vi "Untitled 8 (SubVI).vi"(8 "error in (no error)":errorcluster, 11 "TreeControl in":refnum<vi>) -> (0 "error out":errorcluster, 3 "Setup out":refnum<class "Setup.lvclass">)   [LabVIEW 2013, in "DataCreation.lvlib"]
uses:
  DataCreation.lvlib
  classes/Datastructure/Setup/Setup.lvclass
  classes/Datastructure/Image/img.lvclass
  classes/Datastructure/Device/Device.lvclass
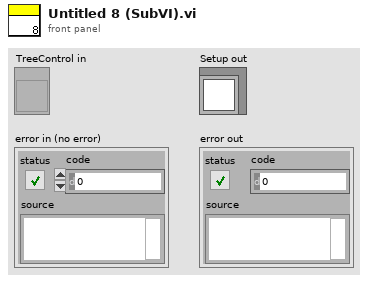
[diagram p1: front panel]
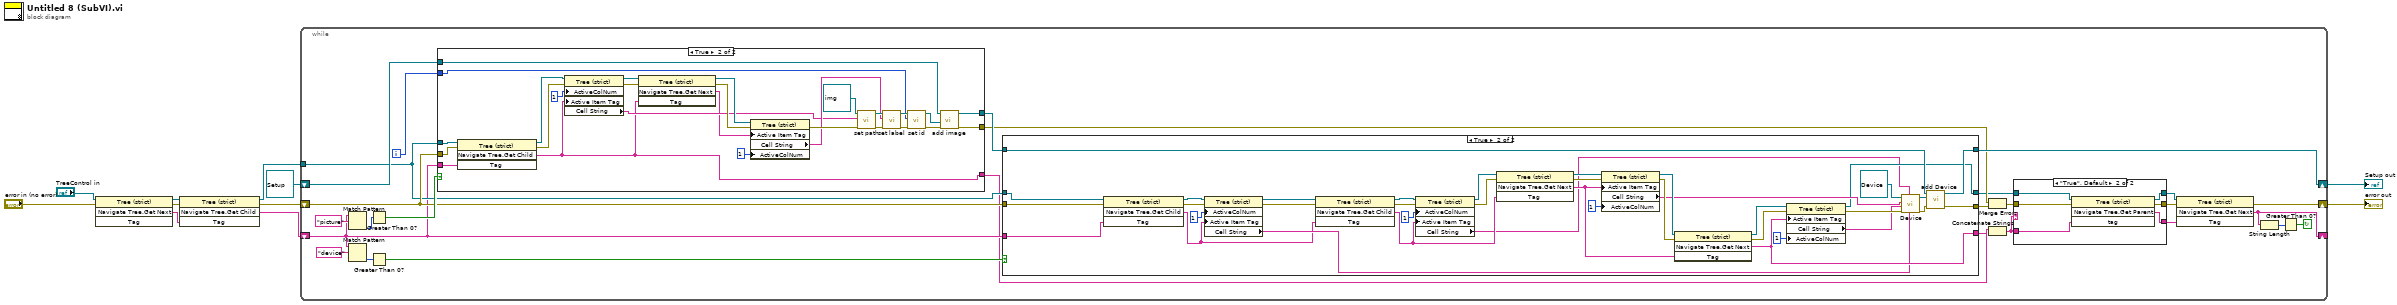
[diagram p0: block diagram]
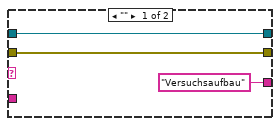
[diagram p2: hidden frame]
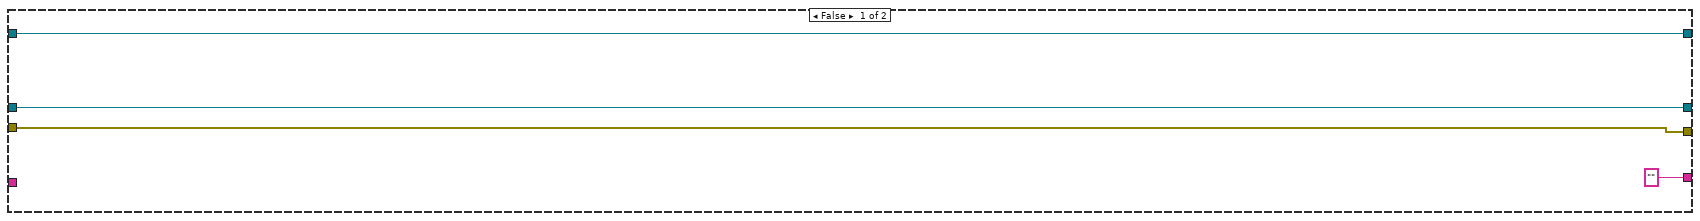
[diagram p3: hidden frame]
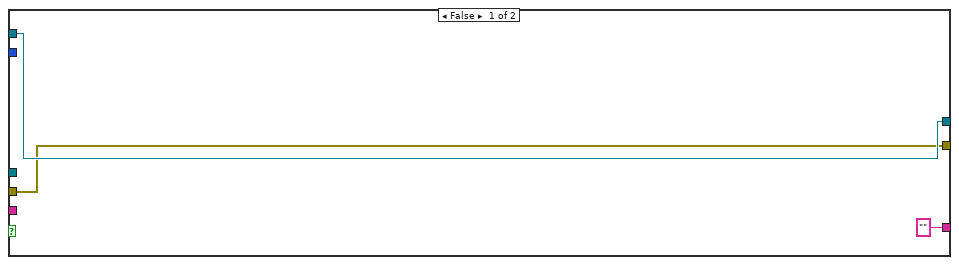
[diagram p4: hidden frame]
diagram:
  n1 = invoke class="Tree (strict)" method="Navigate Tree.Get Next"(reference="TreeControl in", error in="error in (no error)") -> (reference out=w5:refnum<vi>, error out=w6:errorcluster, "Navigate Tree:Get Next Item"=w7:string)  [unwired: 2 in, 1 out]
  n2 = invoke class="Tree (strict)" method="Navigate Tree.Get Child"(reference=w5, error in=w6, "Tag"=w7) -> (reference out=w10:refnum<vi>, error out=w8:errorcluster, "Navigate Tree:Get Child"=w9:string)  [unwired: 1 in, 1 out]
  n3 = while {
    shift-right: [w16] -> w1
    shift-left: w8 -> [w32]
    shift-right: [w25] -> w2
    shift-left: refnum<class "Setup.lvclass"> refnum ("Setup Ausgang") -> [w31]
    shift-right: [w14] -> _
    shift-left: w9 -> [w29]
    tunnel: w10 -> [w30]
    i -> [w12]
    stop <- w19 continue-if-true
    n4 = Match Pattern(string=w29, regular expression="picture" ("Regulärer Ausdruck")) -> (offset past match=w37:i32)  [unwired: 1 in, 3 out]
    n5 = Match Pattern(string=w29, regular expression="device" ("Regulärer Ausdruck")) -> (offset past match=w33:i32)  [unwired: 1 in, 3 out]
    n6 = Greater Than 0?(x=w37) -> (x > 0?=w36:bool)
    n7 = Greater Than 0?(x=w33) -> (x > 0?=w35:bool)
    n8 = case shown="True" w36 {
      tunnel: w29 -> [_ w99]
      tunnel: w32 -> [w89 w100]
      tunnel: w30 -> [_ w101]
      tunnel: [w89 w105] -> w24
      tunnel: w31 -> [w90 w104]
      tunnel: [w90 w98] -> w26
      tunnel: ["" ("Navigate Tree:Get Child") w97] -> w28
      tunnel: w12 -> [_ w94]
      frame False {
      }
      frame True {
        n9 = invoke class="Tree (strict)" method="Navigate Tree.Get Child"(reference=w101, error in=w100, "Tag"=w99) -> (reference out=w103:refnum<vi>, error out=w102:errorcluster, "Navigate Tree:Get Child"=w97:string)  [unwired: 1 in, 1 out]
        n10 = property class="Tree (strict)"(reference=w103, error in=w102, "ActiveColNum"=1 ("Active Cell:Active Column Number"), "Active Item Tag"=w97) -> (reference out=w113:refnum<vi>, error out=w114:errorcluster, "Cell String"=w109:string)
        n11 = invoke class="Tree (strict)" method="Navigate Tree.Get Next"(reference=w113, error in=w114, "Tag"=w97) -> (reference out=w112:refnum<vi>, error out=w111:errorcluster, "Navigate Tree:Get Next Item"=w108:string)  [unwired: 1 in, 1 out]
        n12 = property class="Tree (strict)"(reference=w112, error in=w111, "Active Item Tag"=w108, "ActiveColNum"=1 ("Active Cell:Active Column Number")) -> (error out=w118:errorcluster, "Cell String"=w110:string)  [unwired: 1 out]
        n13 = call-dynamic "set path.vi"("error in (no error)"=w118, "path"=w109, "img (Eingang)"=refnum<class "img.lvclass"> refnum ("img.lvclass")) -> ("error out"=w117:errorcluster, "img (Ausgang)"=w115:refnum<class "img.lvclass">)  [unwired: 7 in]
        n14 = call-dynamic "set label.vi"("error in (no error)"=w117, "label"=w110, "img (Eingang)"=w115) -> ("error out"=w95:errorcluster, "img (Ausgang)"=w96:refnum<class "img.lvclass">)  [unwired: 7 in]
        n15 = call-dynamic "set id.vi"("error in (no error)"=w95, "id"=w94, "img in"=w96) -> ("error out"=w93:errorcluster, "img out"=w92:refnum<class "img.lvclass">)  [unwired: 7 in]
        n16 = call-dynamic "add image.vi"("error in (no error)"=w93, "img.lvclass"=w92, "Setup (Eingang)"=w104) -> ("error out"=w105:errorcluster, "Setup (Ausgang)"=w98:refnum<class "Setup.lvclass">)  [unwired: 7 in]
      }
    }
    n17 = case shown="True" w35 {
      tunnel: w32 -> [w49 w53]
      tunnel: w30 -> [w48 w52]
      tunnel: w29 -> [_ w54]
      tunnel: ["" ("Navigate Tree:Get Next Item") w72] -> w27
      tunnel: w26 -> [w50 w66]
      tunnel: [w49 w67] -> w23
      tunnel: [w50 w65] -> w25
      tunnel: [w48 w64] -> w21
      frame False {
      }
      frame True {
        n18 = invoke class="Tree (strict)" method="Navigate Tree.Get Child"(reference=w52, error in=w53, "Tag"=w54) -> (reference out=w61:refnum<vi>, error out=w60:errorcluster, "Navigate Tree:Get Child"=w55:string)  [unwired: 1 in, 1 out]
        n19 = property class="Tree (strict)"(reference=w61, error in=w60, "ActiveColNum"=1 ("Active Cell:Active Column Number"), "Active Item Tag"=w55) -> (reference out=w57:refnum<vi>, error out=w58:errorcluster, "Cell String"=w56:string)
        n20 = invoke class="Tree (strict)" method="Navigate Tree.Get Child"(reference=w57, error in=w58, "Tag"=w55) -> (reference out=w81:refnum<vi>, error out=w82:errorcluster, "Navigate Tree:Get Child"=w80:string)  [unwired: 1 in, 1 out]
        n21 = property class="Tree (strict)"(reference=w81, error in=w82, "ActiveColNum"=1 ("Active Cell:Active Column Number"), "Active Item Tag"=w80) -> (reference out=w87:refnum<vi>, error out=w88:errorcluster, "Cell String"=w62:string)
        n22 = invoke class="Tree (strict)" method="Navigate Tree.Get Next"(reference=w87, error in=w88, "Tag"=w80) -> (reference out=w86:refnum<vi>, error out=w85:errorcluster, "Navigate Tree:Get Next Item"=w73:string)  [unwired: 1 in, 1 out]
        n23 = property class="Tree (strict)"(reference=w86, error in=w85, "Active Item Tag"=w73, "ActiveColNum"=1 ("Active Cell:Active Column Number")) -> (reference out=w78:refnum<vi>, error out=w79:errorcluster, "Cell String"=w74:string)
        n24 = invoke class="Tree (strict)" method="Navigate Tree.Get Next"(reference=w78, error in=w79, "Tag"=w73) -> (reference out=w77:refnum<vi>, error out=w76:errorcluster, "Navigate Tree:Get Next Item"=w72:string)  [unwired: 1 in, 1 out]
        n25 = property class="Tree (strict)"(reference=w77, error in=w76, "Active Item Tag"=w72, "ActiveColNum"=1 ("Aktive Zelle:Nummer der aktiven Spalte")) -> (reference out=w64:refnum<vi>, error out=w71:errorcluster, "Cell String"=w63:string)
        n26 = call-dynamic "Device.vi"("Model"=w56, "last calibration"=w62, "error in (no error)"=w71, "Hersteller"=w63, "serial"=w74, "Device Eingang"=refnum<class "Device.lvclass"> refnum ("Device.lvclass")) -> ("error out"=w68:errorcluster, "Device Ausgang"=w69:refnum<class "Device.lvclass">)  [unwired: 4 in]
        n27 = call-dynamic "add Device.vi"("error in (no error)"=w68, "Device.lvclass"=w69, "Setup Eingang"=w66) -> ("error out"=w67:errorcluster, "Setup Ausgang"=w65:refnum<class "Setup.lvclass">)  [unwired: 7 in]
      }
    }
    n28 = Merge Errors(w24, w23) -> (w22:errorcluster)
    n29 = Concatenate Strings(w28, w27) -> (w13:string)
    n30 = case shown="\"True\", Default" w13 {
      tunnel: w22 -> [w41 w47]
      tunnel: w21 -> [w40 w46]
      tunnel: w13 -> [_ w45]
      tunnel: [w41 w44] -> w18
      tunnel: [w40 w43] -> w17
      tunnel: ["Versuchsaufbau" ("Navigate Tree:Get Parent") w42] -> w15
      frame "" {
      }
      frame "True", Default {
        n31 = invoke class="Tree (strict)" method="Navigate Tree.Get Parent"(reference=w46, error in=w47, "tag"=w45) -> (reference out=w43:refnum<vi>, error out=w44:errorcluster, "Navigate Tree:Get Parent"=w42:string)  [unwired: 1 in, 1 out]
      }
    }
    n32 = invoke class="Tree (strict)" method="Navigate Tree.Get Next"(reference=w17, error in=w18, "Tag"=w15) -> (error out=w16:errorcluster, "Navigate Tree:Get Next Item"=w14:string)  [unwired: 1 in, 2 out]
    n33 = String Length(string=w14) -> (length=w20:i32)
    n34 = Greater Than 0?(x=w20) -> (x > 0?=w19:bool)
  }
  "Setup out" <- w2
  "error out" <- w1
